vi "SubVI_Save_Survey.vi"(8 "error in (no error)":errorcluster) -> (0 "error out":errorcluster)   [LabVIEW 2020]
uses:
  Global 1.vi
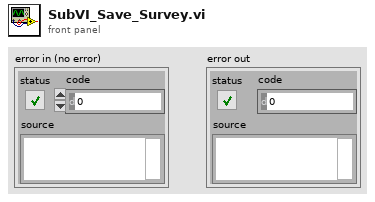
[diagram p1: front panel]
types:
  T1 = enum16{"open", "open or create", "create or replace", "create", "open (read-only)"}
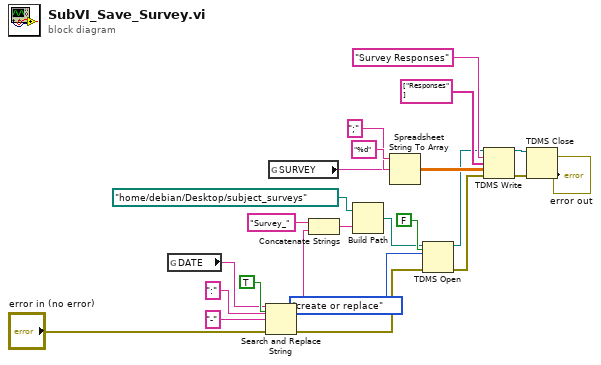
[diagram p0: block diagram]
diagram:
  n1 = global read "Global 1.vi" "DATE"() -> (w5:string)
  n2 = Search and Replace String(replace all?=TRUE ("replace all? (F)"), input string=w5, search string=":" ("input string"), replace string="-" ("replace string (\"\")"), error in="error in (no error)") -> (result string=w4:string, error out=w14:errorcluster)  [unwired: 3 in, 2 out]
  n3 = global read "Global 1.vi" "SURVEY"() -> (w18:string)
  n4 = Concatenate Strings("Survey_" ("string"), w4) -> (w8:string)
  n5 = Build Path(base path=path "/home/debian/Desktop/subject_surveys", name or relative path=w8) -> (appended path=w17:path)
  n6 = Spreadsheet String To Array(delimiter (Tab)=";", format string="%d", spreadsheet string=w18) -> (array=w24:dbl[][])  [unwired: 1 in]
  n7 = TDMS Open(5:FALSE ("create index file? (T)"), 8:w14, 10:T1."create or replace" ("operation (0:open)"), 11:w17) -> (0:w12:errorcluster, 3:w11:refnum<k34>)  [unwired: 3 in]
  n8 = TDMS Write(0:w11, 5:"Survey Responses" ("channel name(s) in (Untitled)"), 7:string[] ["Responses"] ("channel name(s) in (Untitled)"), 9:w24, 11:w12) -> (4:w10:refnum<k34>, 15:w13:errorcluster)  [unwired: 1 in, 2 out]
  n9 = TDMS Close(8:w13, 11:w10) -> (0:→"error out":errorcluster)  [unwired: 1 out]
